vi "WIN10 BLE Test.vi"() -> ()   [LabVIEW 2015]
uses:
  user32.dll
  Touch Monitoring/tchdbg.dll
  C:/Windows/System32/BluetoothApis.dll
  C:/Windows/System32/setupapi.dll
panel:
  out "return type":i32
  out "hDevice":i64
  out "Data":i8[](array[numeric])
  out "반환 타입":i32
  in  "Window Name":string
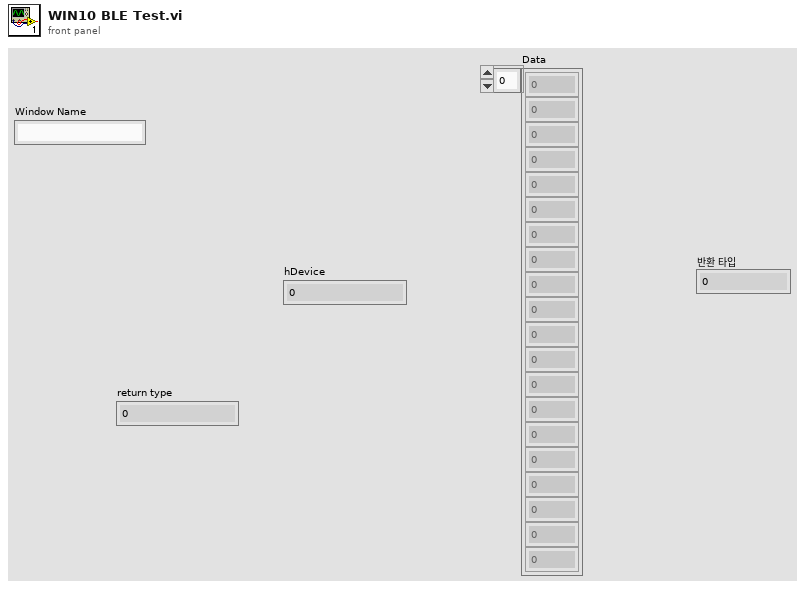
[diagram p1: front panel]
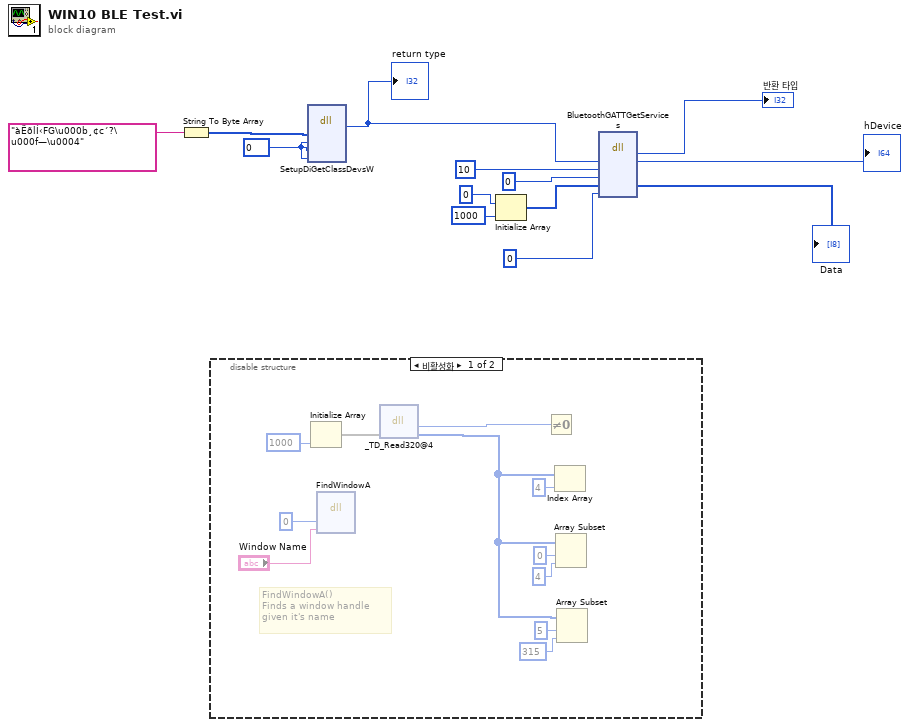
[diagram p0: block diagram]
diagram:
  w2 = i8 0 ("index")
  n1 = String To Byte Array(string="àËðlÍ‹FG\u000b¸¢c´?\u000f—\u0004") -> (unsigned byte array=w3:u8[])
  n2 = disable-structure shown="비활성화" {
    frame Disabled {
      # "FindWindowA()\nFinds a window handle \ngiven it's name"
      n3 = Initialize Array(1000 ("dimension size")) -> (w23:void[])  [unwired: 1 in]
      n4 = dll-call lib="user32.dll" fn="FindWindowA"("arg1"=0, "arg2"="Window Name") -> ()  [unwired: 4 in, 4 out]
      n5 = dll-call lib="C:/Users/im tech/Desktop/Touch Monitoring/tchdbg.dll" fn="_TD_Read320@4" label="TD_Read320"("Buf"=w23) -> ("반환 타입"=w21:i32, "Buf"=w16:i8[])  [unwired: 3 in, 2 out]
      n6 = Not Equal To 0?(x=w21) -> ()  [unwired: 1 out]
      n7 = Index Array(array=w16, index=4 ("인덱스")) -> ()  [unwired: 1 out]
      n8 = Array Subset(array=w16, index=0 ("인덱스"), length=4 ("인덱스")) -> ()  [unwired: 1 out]
      n9 = Array Subset(array=w16, index=5 ("인덱스"), length=315 ("인덱스")) -> ()  [unwired: 1 out]
    }
    frame Enabled {
    }
  }
  n10 = dll-call lib="C:/Windows/System32/setupapi.dll" fn="SetupDiGetClassDevsW"("ClassGuid"=w3, "Enum"=w2, "hwndParent"=w2, "Falgs"=w2) -> ("return type"=w1:i32)  [unwired: 4 in, 5 out]
  "return type" <- w1
  n11 = Initialize Array(i8 0 ("index"), 1000 ("dimension size")) -> (w10:i8[])
  n12 = dll-call lib="C:/Windows/System32/BluetoothApis.dll" fn="BluetoothGATTGetServices"("hDevice"=w1, "Cnt"=i8 10 ("index"), "Buf"=i8 0 ("index"), "Data"=w10, "Flag"=i8 0 ("index")) -> ("반환 타입"=→"반환 타입":i32, "hDevice"=→"hDevice":i64, "Data"=→"Data":i8[])  [unwired: 6 in, 2 out]
